vi "append.vi"(7 "add mode":T1=enum."copy", 8 "error in (no error)":errorcluster, 10 "Image.lvclass":refnum<class "Image.lvclass">, 11 "ImageCollection in":refnum<class "ImageCollection.lvclass">) -> (0 "error out":errorcluster, 2 "new number of images":i32, 3 "ImageCollection out":refnum<class "ImageCollection.lvclass">)   [LabVIEW 2010, in "ImageCollection.lvclass"]
uses:
  ImageCollection.lvclass
  Image/Image/Image.lvclass
  add_mode_enum.ctl
  Image/Image/storage_mode.ctl
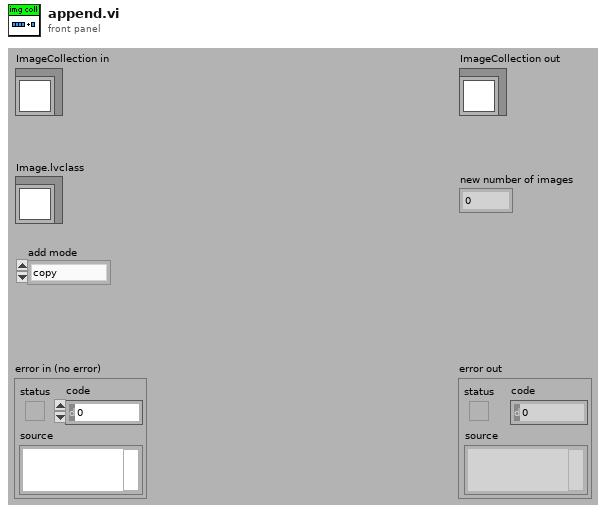
[diagram p1: front panel]
types:
  T1 = typedef "ImageCollection.lvclass/add_mode_enum.ctl" = enum16{"instance", "copy"}
  T2 = typedef "Image.lvclass/storage_mode.ctl" = enum16{"RAM", "disk"}
  T3 = typedef "ImageCollection.lvclass/storage_mode_enum.ctl" = enum16{"RAM", "single files", "multipage TIFF (read-only)"}
  T4 = typedef "Image Type" = u32
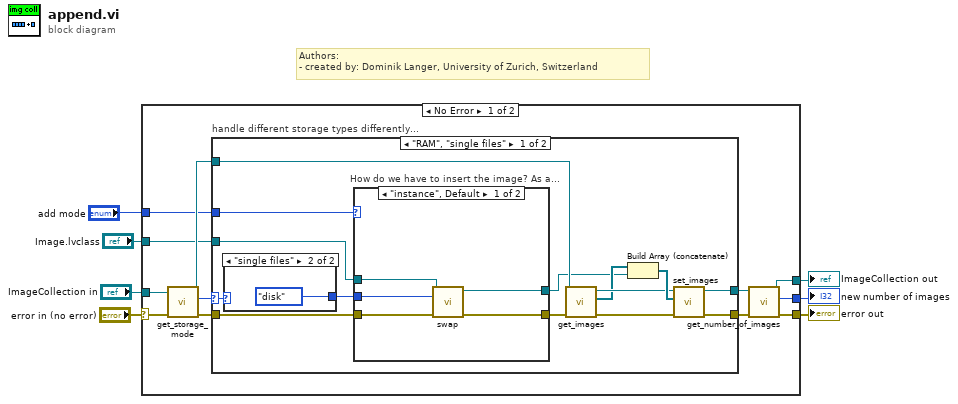
[diagram p0: block diagram]
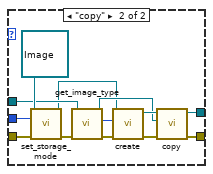
[diagram p2: hidden frame]
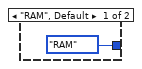
[diagram p3: hidden frame]
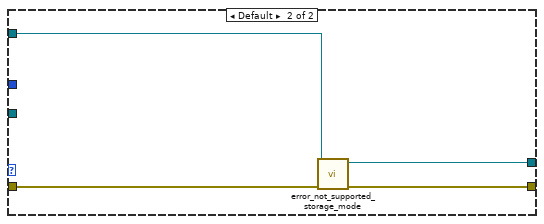
[diagram p4: hidden frame]
diagram:
  # "Authors: \n- created by: Dominik Langer, University of Zurich, Switzerland"
  n1 = case shown="No Error" "error in (no error)" {
    selector: "error in (no error)" -> [w14 w59]
    tunnel: [w18 w59] -> w6
    tunnel: [w16 w58] -> w4
    tunnel: "ImageCollection in" -> [w13 w58]
    tunnel: "Image.lvclass" -> [w9 _]
    tunnel: "add mode" -> [w8 _]
    tunnel: [w15 _] -> w1
    frame No Error {
      n2 = call-dynamic "get_storage_mode.vi"("error in (no error)"=w14, "ImageCollection.lvclass in"=w13) -> ("error out"=w11:errorcluster, "storage type"=w10:T3, "ImageCollection.lvclass out"=w12:refnum<class "ImageCollection.lvclass">)  [unwired: 7 out]
      n3 = case "handle different storage types differently..." shown="\"RAM\", \"single files\"" w10 {
        selector: w10 -> [w33 _]
        tunnel: w11 -> [w25 w57]
        tunnel: [w30 w56] -> w19
        tunnel: w12 -> [w28 w55]
        tunnel: [w31 w54] -> w17
        tunnel: w9 -> [w23 _]
        tunnel: w8 -> [w21 _]
        frame "RAM", "single files" {
          n4 = case shown="\"single files\"" w33 {
            tunnel: [storage_mode."RAM" ("storage type target") storage_mode."disk" ("storage type target")] -> w24
            frame "RAM", Default {
            }
            frame "single files" {
            }
          }
          n5 = case "How do we have to insert the image? As a..." shown="\"instance\", Default" w21 {
            tunnel: [w37 w51] -> w22
            tunnel: [w35 w50] -> w20
            tunnel: w25 -> [w38 w45]
            tunnel: w24 -> [w36 w42]
            tunnel: w23 -> [w34 w41]
            frame "instance", Default {
              n6 = call-dynamic "swap.vi"("error in (no error)"=w38, "storage type target"=w36, "Image in"=w34) -> ("error out"=w37:errorcluster, "Image out"=w35:refnum<class "Image.lvclass">)  [unwired: 7 out]
            }
            frame "copy" {
              n7 = call-dynamic "set_storage_mode.vi"("error in (no error)"=w45, "storage type"=w42, "Image.lvclass in"=refnum<class "Image.lvclass"> refnum ("Image.lvclass")) -> ("error out"=w44:errorcluster, "Image.lvclass out"=w39:refnum<class "Image.lvclass">)  [unwired: 7 out]
              n8 = call-dynamic "get_image_type.vi"("error in (no error)"=w44, "Image.lvclass in"=w41) -> ("error out"=w49:errorcluster, "Image Type"=w48:T4, "Image.lvclass out"=w40:refnum<class "Image.lvclass">)  [unwired: 7 out]
              n9 = call "create.vi"("error in (no error)"=w49, "Image Type"=w48, "Image in"=w39) -> ("error out"=w46:errorcluster, "Image out"=w47:refnum<class "Image.lvclass">)  [unwired: 1 in, 6 out]
              n10 = call "copy.vi"("error in (no error)"=w46, "image to copy (source)"=w40, "Image in (target)"=w47) -> ("error out"=w51:errorcluster, "Image out"=w50:refnum<class "Image.lvclass">)  [unwired: 7 out]
            }
          }
          n11 = call-dynamic "get_images.vi"("error in (no error)"=w22, "ImageCollection.lvclass in"=w28) -> ("error out"=w29:errorcluster, "images"=w26:refnum<class "Image.lvclass">[], "ImageCollection.lvclass out"=w27:refnum<class "ImageCollection.lvclass">)  [unwired: 7 out]
          n12 = Build Array (concatenate)(w26, w20) -> (w32:refnum<class "Image.lvclass">[])
          n13 = call-dynamic "set_images.vi"("error in (no error)"=w29, "images"=w32, "ImageCollection.lvclass in"=w27) -> ("error out"=w30:errorcluster, "ImageCollection.lvclass out"=w31:refnum<class "ImageCollection.lvclass">)  [unwired: 7 out]
        }
        frame Default {
          n14 = call-dynamic "error_not_supported_storage_mode.vi"("error in (no error)"=w57, "ImageCollection in"=w55) -> ("error out"=w56:errorcluster, "ImageCollection out"=w54:refnum<class "ImageCollection.lvclass">)  [unwired: 8 out]
        }
      }
      n15 = call-dynamic "get_number_of_images.vi"("error in (no error)"=w19, "ImageCollection in"=w17) -> ("error out"=w18:errorcluster, "size"=w15:i32, "ImageCollection out"=w16:refnum<class "ImageCollection.lvclass">)  [unwired: 7 out]
    }
    frame Error {
    }
  }
  "error out" <- w6
  "ImageCollection out" <- w4
  "new number of images" <- w1
